vi "Introduction Demo_Global_OnCommand.vi"(10 "Command ID":string, 11 "Object":T1) -> ()   [LabVIEW 2015]
uses:
  <resource>/Framework/Providers/API/ItemRef.ctl
panel:
  out "error out":errorcluster
  in  "error in":errorcluster
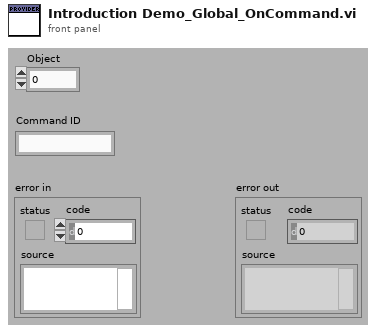
[diagram p1: front panel]
types:
  T1 = typedef "ItemRef.ctl" = u64
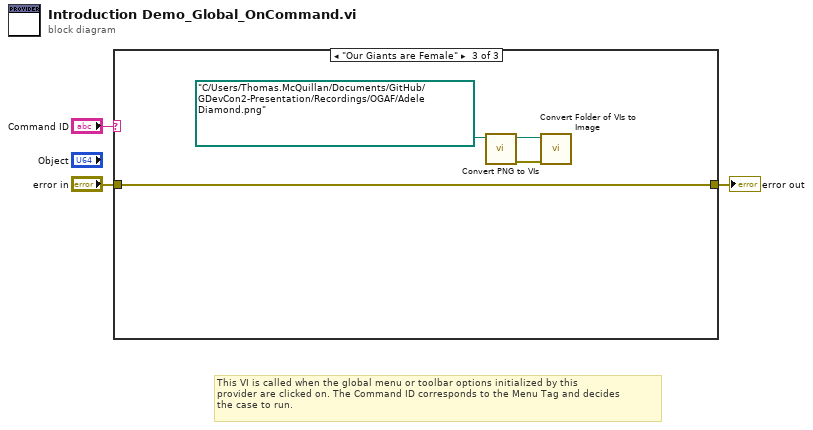
[diagram p0: block diagram]
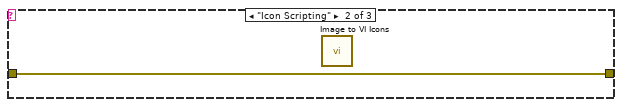
[diagram p3: hidden frame]
diagram:
  # "This VI is called when the global menu or toolbar options initialized by this \nprovider are clicked on. The Command ID corresponds to the Menu Tag and decides\nthe case to run."
  n1 = case shown="\"Our Giants are Female\"" "Command ID" {
    tunnel: "error in" -> [w4 w5 w6]
    tunnel: [w4 w5 w6] -> w1
    frame Default {
    }
    frame "Icon Scripting" {
      n2 = call <resource>:"Image to VI Icons.vi"() -> ()  [unwired: 12 in]
    }
    frame "Our Giants are Female" {
      n3 = call <resource>:"Convert PNG to VIs.vi"("selected path"=path "C:/Users/Thomas.McQuillan/Documents/GitHub/GDevCon2-Presentation/Recordings/OGAF/Adele Diamond.png") -> ("error out"=w9:errorcluster, "directory copy"=w8:path)  [unwired: 9 in]
      n4 = call <resource>:"Convert Folder of VIs to Image.vi"("error in (no error)"=w9, "Folder Path"=w8) -> ()  [unwired: 9 in, 1 out]
    }
  }
  "error out" <- w1
